vi "Save As Raw.vi"(8 "error in (no error)":errorcluster, 10 "typ":i32, 11 "szFileTitle":string) -> (0 "error out":errorcluster, 2 "function return":u32, 3 "szFileTitle out":string)   [LabVIEW 2014, in "atmcd32d.lvlib"]
doc: "unsigned int WINAPI SaveAsRaw(char * szFileTitle, int typ);"
uses:
  atmcd32d.lvlib
  atmcd32d.dll
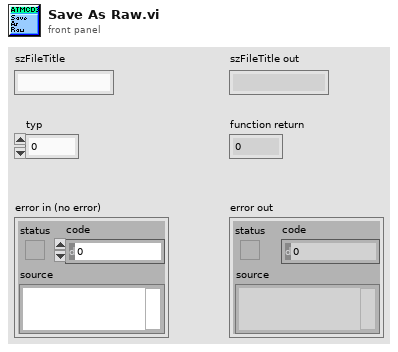
[diagram p1: front panel]
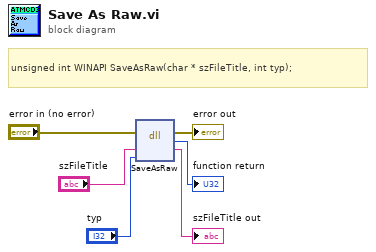
[diagram p0: block diagram]
diagram:
  # "unsigned int WINAPI SaveAsRaw(char * szFileTitle, int typ);"
  n1 = dll-call lib="C:/Users/Bakir/Documents/Lambda2-Testing/lib/Andorlib/atmcd32d.*" fn="SaveAsRaw"(error in="error in (no error)", "szFileTitle"="szFileTitle", "typ"="typ") -> (error out=→"error out":errorcluster, →"function return":u32, "szFileTitle"=→"szFileTitle out":string)  [unwired: 3 in, 1 out]
